vi "Installer.vi"() -> ()   [LabVIEW 2014]
panel:
  out "This Version Date":string
  out "This Version":string
  out "Installed Version Date":string
  out "Installed Version":string
  out "Installation Path":path
  in  "Deinstall Button":bool
  in  "Cancel Button":bool
  in  "Install Button":bool
  # "This VI installes the CSPP_Message Maker into the default LabVIEW directory.\nBelow are information about the current installation as well as this installation:"
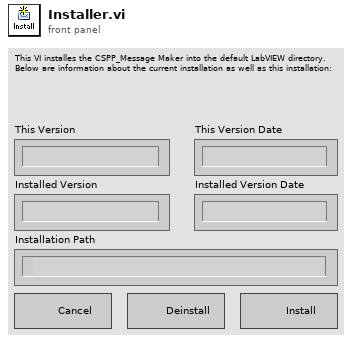
[diagram p1: front panel]
types:
  T1 = enum16{"open", "replace", "create", "open or create", "replace or create", "replace or create with confirmation"}
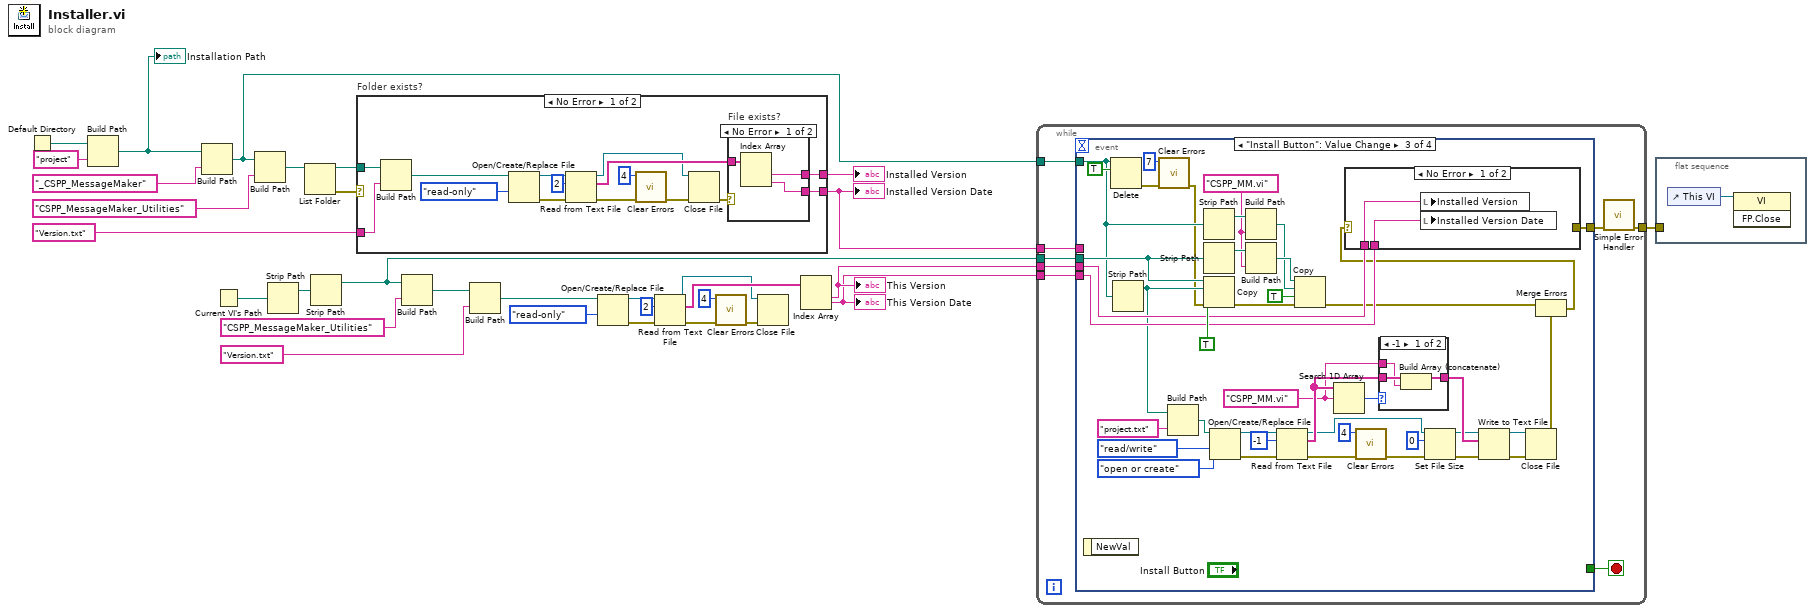
[diagram p0: block diagram]
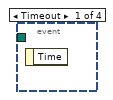
[diagram p2: hidden frame]
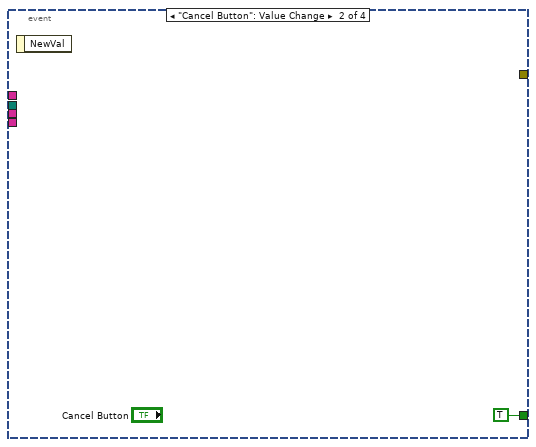
[diagram p3: hidden frame]
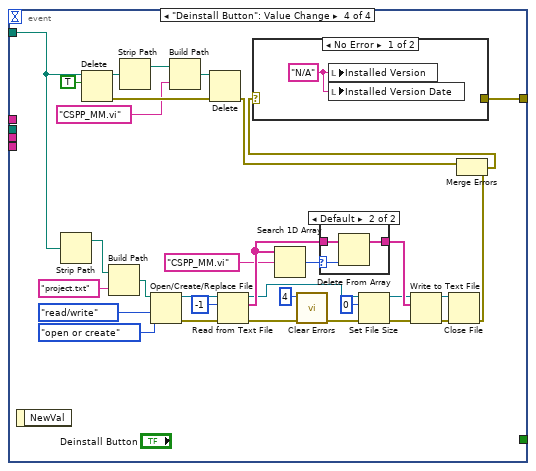
[diagram p6: hidden frame]
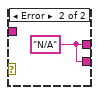
[diagram p9: hidden frame]
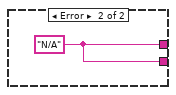
[diagram p10: hidden frame]
diagram:
  n1 = Default Directory() -> (w31:path)
  n2 = Build Path(base path=w31, name or relative path="project") -> (appended path=w23:path)
  "Installation Path" <- w23
  n3 = Build Path(base path=w23, name or relative path="_CSPP_MessageMaker") -> (appended path=w7:path)
  n4 = Current VI's Path() -> (path=w21:path)
  n5 = Build Path(base path=w7, name or relative path="CSPP_MessageMaker_Utilities") -> (appended path=w26:path)
  n6 = Strip Path(path=w21) -> (stripped path=w11:path)  [unwired: 1 out]
  n7 = List Folder(path=w26) -> (path out=w25:path, error out=w24:errorcluster)  [unwired: 3 in, 2 out]
  n8 = Strip Path(path=w11) -> (stripped path=w5:path)  [unwired: 1 out]
  n9 = case "Folder exists?" shown="No Error" w24 {
    tunnel: "Version.txt" ("name or relative path") -> [w46 _]
    tunnel: w25 -> [w40 _]
    tunnel: [w37 w51] -> w22
    tunnel: [w36 w51] -> w10
    frame No Error {
      n10 = Build Path(base path=w40, name or relative path=w46) -> (appended path=w45:path)
      n11 = Open/Create/Replace File(file path (use dialog)=w45, access (0:read/write)=enum16{"read/write", "read-only", "write-only"}."read-only") -> (refnum out=w43:refnum<file>, error out=w42:errorcluster)  [unwired: 4 in, 1 out]
      n12 = Read from Text File(file (use dialog)=w43, count=2, error in=w42) -> (refnum out=w32:refnum<file>, text=w38:string[], error out=w33:errorcluster)  [unwired: 1 in, 1 out]
      n13 = call <vilib>:"Clear Errors.vi"("error in (no error)"=w33, "specific error code to clear (0: all)"=4) -> ("error out"=w34:errorcluster)  [unwired: 4 in, 1 out]
      n14 = Close File(refnum=w32, error in=w34) -> (error out=w39:errorcluster)  [unwired: 1 out]
      n15 = case "File exists?" shown="No Error" w39 {
        tunnel: w38 -> [w49 _]
        tunnel: [w48 w50] -> w37
        tunnel: [w47 w50] -> w36
        frame No Error {
          n16 = Index Array(array=w49) -> (element #1=w48:string, element #2=w47:string)  [unwired: 2 in]
        }
        frame Error {
          w50 = "N/A"
        }
      }
    }
    frame Error {
      w51 = "N/A"
    }
  }
  "Installed Version" <- w22
  "Installed Version Date" <- w10
  n17 = Build Path(base path=w5, name or relative path="CSPP_MessageMaker_Utilities") -> (appended path=w14:path)
  n18 = Build Path(base path=w14, name or relative path="Version.txt") -> (appended path=w19:path)
  n19 = Open/Create/Replace File(file path (use dialog)=w19, access (0:read/write)=enum16{"read/write", "read-only", "write-only"}."read-only") -> (refnum out=w17:refnum<file>, error out=w16:errorcluster)  [unwired: 4 in, 1 out]
  n20 = Read from Text File(file (use dialog)=w17, count=2, error in=w16) -> (refnum out=w1:refnum<file>, text=w12:string[], error out=w3:errorcluster)  [unwired: 1 in, 1 out]
  n21 = call <vilib>:"Clear Errors.vi"("error in (no error)"=w3, "specific error code to clear (0: all)"=4) -> ("error out"=w2:errorcluster)  [unwired: 4 in, 1 out]
  n22 = Close File(refnum=w1, error in=w2) -> ()  [unwired: 2 out]
  n23 = Index Array(array=w12) -> (element #1=w9:string, element #2=w8:string)  [unwired: 2 in]
  "This Version" <- w9
  "This Version Date" <- w8
  n24 = while {
    tunnel: w10 -> [w59]
    tunnel: w9 -> [w58]
    tunnel: w8 -> [w56]
    tunnel: w7 -> [w55]
    tunnel: [w53] -> w6
    tunnel: w5 -> [w52]
    stop <- w57 stop-if-true
    n25 = event shown="[2] \"Install Button\": Value Change" {
      selector: _ -> [_ _ _ _]
      dyn-events: _ -> [_ _ _ _]
      timeout: _ -> [_ _ _ _]
      tunnel: w59 -> [_ _ _ _]
      tunnel: w58 -> [_ _ w90 _]
      tunnel: [_ TRUE _ _] -> w57
      tunnel: w56 -> [_ _ w91 _]
      tunnel: w55 -> [_ _ w64 w118]
      tunnel: [_ _ w92 w134] -> w54
      tunnel: w52 -> [_ _ w99 _]
      event Timeout {
        n26 = event-data() -> ()  [unwired: 1 in, 1 out]
      }
      event "Cancel Button": Value Change {
        n27 = event-data() -> ()  [unwired: 1 in, 1 out]
      }
      event "Install Button": Value Change {
        w74 = "CSPP_MM.vi" ("element")
        w96 = "CSPP_MM.vi" ("name or relative path")
        n28 = event-data() -> ()  [unwired: 1 in, 1 out]
        n29 = Delete(path (use dialog)=w64, entire hierarchy (F)=TRUE) -> (error out=w62:errorcluster)  [unwired: 3 in, 2 out]
        n30 = Strip Path(path=w64) -> (stripped path=w75:path)  [unwired: 1 out]
        n31 = call <vilib>:"Clear Errors.vi"("error in (no error)"=w62, "specific error code to clear (0: all)"=7) -> ("error out"=w61:errorcluster)  [unwired: 4 in, 1 out]
        n32 = Build Path(base path=w75, name or relative path="project.txt") -> (appended path=w82:path)
        n33 = Strip Path(path=w64) -> (stripped path=w98:path)  [unwired: 1 out]
        n34 = Strip Path(path=w99) -> (stripped path=w97:path)  [unwired: 1 out]
        n35 = Copy(8:w61, 9:TRUE ("overwrite (F)"), 10:w75, 11:w99) -> (0:w101:errorcluster)  [unwired: 1 in, 2 out]
        n36 = Open/Create/Replace File(file path (use dialog)=w82, operation (0:open)=T1."open or create", access (0:read/write)=enum16{"read/write", "read-only", "write-only"}."read/write") -> (refnum out=w79:refnum<file>, error out=w78:errorcluster)  [unwired: 3 in, 1 out]
        n37 = Build Path(base path=w98, name or relative path=w96) -> (appended path=w94:path)
        n38 = Build Path(base path=w97, name or relative path=w96) -> (appended path=w95:path)
        n39 = Read from Text File(file (use dialog)=w79, count=-1, error in=w78) -> (refnum out=w69:refnum<file>, text=w87:string[], error out=w80:errorcluster)  [unwired: 1 in, 1 out]
        n40 = Copy(8:w101, 9:TRUE ("overwrite (F)"), 10:w94, 11:w95) -> (0:w68:errorcluster)  [unwired: 1 in, 2 out]
        n41 = Search 1D Array(1D array=w87, element=w74) -> (index of element=w89:i32)  [unwired: 1 in]
        n42 = call <vilib>:"Clear Errors.vi"("error in (no error)"=w80, "specific error code to clear (0: all)"=4) -> ("error out"=w70:errorcluster)  [unwired: 4 in, 1 out]
        n43 = case shown="-1" w89 {
          tunnel: w87 -> [w104 w105]
          tunnel: [w103 w105] -> w88
          tunnel: w74 -> [w102 _]
          frame -1 {
            n44 = Build Array (concatenate)(w104, w102) -> (w103:string[])
          }
          frame Default {
          }
        }
        n45 = Set File Size(4:w70, 6:i64 0 ("size (in bytes)"), 7:w69) -> (0:w72:errorcluster, 3:w71:refnum<file>)
        n46 = Write to Text File(file (use dialog)=w71, text=w88, error in=w72) -> (refnum out=w85:refnum<file>, error out=w84:errorcluster)  [unwired: 1 in, 1 out]
        n47 = Close File(refnum=w85, error in=w84) -> (error out=w67:errorcluster)  [unwired: 1 out]
        n48 = Merge Errors(w68, w67) -> (w66:errorcluster)
        n49 = case shown="No Error" w66 {
          selector: w66 -> [_ w108]
          tunnel: [_ w108] -> w92
          tunnel: w91 -> [w107 _]
          tunnel: w90 -> [w106 _]
          frame No Error {
            n50 = local write "Installed Version"(w106) -> ()
            n51 = local write "Installed Version Date"(w107) -> ()
          }
          frame Error {
          }
        }
      }
      event "Deinstall Button": Value Change {
        n52 = event-data() -> ()  [unwired: 1 in, 1 out]
        n53 = Strip Path(path=w118) -> (stripped path=w117:path)  [unwired: 1 out]
        n54 = Delete(path (use dialog)=w118, entire hierarchy (F)=TRUE) -> (deleted path=w139:path, error out=w138:errorcluster)  [unwired: 3 in, 1 out]
        n55 = Build Path(base path=w117, name or relative path="project.txt") -> (appended path=w125:path)
        n56 = Strip Path(path=w139) -> (stripped path=w136:path)  [unwired: 1 out]
        n57 = Open/Create/Replace File(file path (use dialog)=w125, operation (0:open)=T1."open or create", access (0:read/write)=enum16{"read/write", "read-only", "write-only"}."read/write") -> (refnum out=w122:refnum<file>, error out=w121:errorcluster)  [unwired: 3 in, 1 out]
        n58 = Build Path(base path=w136, name or relative path="CSPP_MM.vi") -> (appended path=w137:path)
        n59 = Delete(path (use dialog)=w137, error in=w138) -> (error out=w110:errorcluster)  [unwired: 3 in, 2 out]
        n60 = Read from Text File(file (use dialog)=w122, count=-1, error in=w121) -> (refnum out=w113:refnum<file>, text=w131:string[], error out=w123:errorcluster)  [unwired: 1 in, 1 out]
        n61 = Search 1D Array(1D array=w131, element="CSPP_MM.vi") -> (index of element=w133:i32)  [unwired: 1 in]
        n62 = call <vilib>:"Clear Errors.vi"("error in (no error)"=w123, "specific error code to clear (0: all)"=4) -> ("error out"=w116:errorcluster)  [unwired: 4 in, 1 out]
        n63 = case shown="Default" w133 {
          selector: w133 -> [_ w142]
          tunnel: w131 -> [w141 w144]
          tunnel: [w141 w143] -> w132
          frame -1 {
          }
          frame Default {
            n64 = Delete From Array(array=w144, index=w142) -> (array with subset deleted=w143:string[])  [unwired: 1 in, 1 out]
          }
        }
        n65 = Set File Size(4:w116, 6:i64 0 ("size (in bytes)"), 7:w113) -> (0:w115:errorcluster, 3:w114:refnum<file>)
        n66 = Write to Text File(file (use dialog)=w114, text=w132, error in=w115) -> (refnum out=w128:refnum<file>, error out=w127:errorcluster)  [unwired: 1 in, 1 out]
        n67 = Close File(refnum=w128, error in=w127) -> (error out=w111:errorcluster)  [unwired: 1 out]
        n68 = Merge Errors(w110, w111) -> (w109:errorcluster)
        n69 = case shown="No Error" w109 {
          selector: w109 -> [_ w146]
          tunnel: [_ w146] -> w134
          frame No Error {
            w145 = "N/A" ("Installed Version")
            n70 = local write "Installed Version"(w145) -> ()
            n71 = local write "Installed Version Date"(w145) -> ()
          }
          frame Error {
          }
        }
      }
    }
    n72 = call <vilib>:"Simple Error Handler.vi"("error in (no error)"=w54) -> ("error out"=w53:errorcluster)  [unwired: 4 in, 4 out]
  }
  n73 = flat-sequence {
    tunnel: w6 -> [_]
    frame #0 {
      n74 = control-ref of="This VI"() -> (w147:refnum<vi>)
      n75 = invoke class="VI" method="FP.Close"(reference=w147) -> ()  [unwired: 2 in, 3 out]
    }
  }
